vi "Update Dynamic Configurations.vi"(8 "error in":errorcluster, 10 "AsyncRequest":T2, 11 "Compiled.Settings in":T1) -> (0 "error out":errorcluster, 2 "Response Ref":refnum<queue>, 3 "Compiled.Settings out":T1)   [LabVIEW 2025, in "Runtime Configuration Support Inline Async Example Engine.lvlib"]
uses:
  Runtime Configuration Support Inline Async Example Engine.lvlib
  Shared/Compiled.Settings.ctl
  Shared/AsyncRequest.ctl
  Shared/Runtime Configuration Support Inline Async Example Shared.lvlib
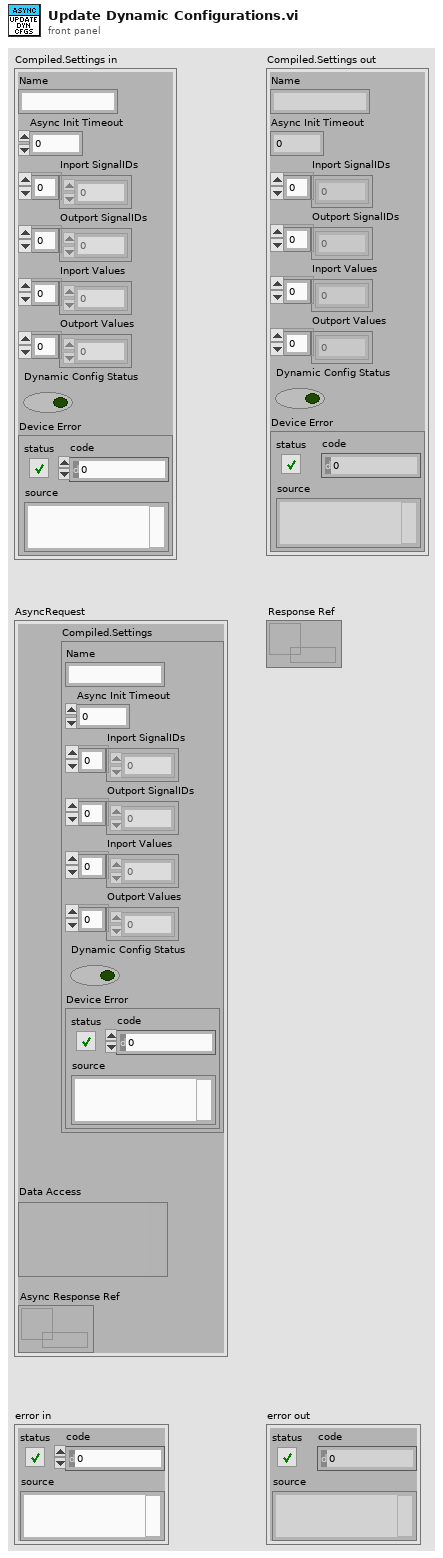
[diagram p1: front panel]
types:
  T1 = typedef "Runtime Configuration Support Inline Async Example Shared.lvlib/Compiled.Settings.ctl" = cluster{"Name":string, "Async Init Timeout":u16, "Inport SignalIDs":i32[], "Outport SignalIDs":i32[], "Inport Values":dbl[], "Outport Values":dbl[], "Dynamic Config Status":bool, "Device Error":errorcluster}
  T2 = typedef "Runtime Configuration Support Inline Async Example Engine.lvlib/AsyncRequest.ctl" = cluster{"Compiled.Settings":T1, "Data Access":variant, "Async Response Ref":refnum<queue>}
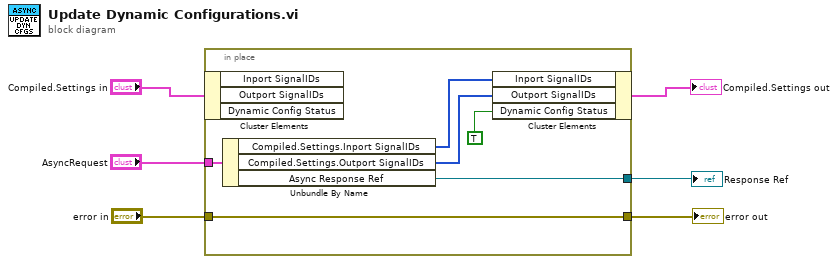
[diagram p0: block diagram]
diagram:
  n1 = in-place {
    in-place-border: "AsyncRequest" -> [w11]
    in-place-border: [w8] -> w2
    in-place-border: "error in" -> [w12]
    in-place-border: [w12] -> w5
    n2 = in-place-cluster #1("Compiled.Settings in") -> ()  [unwired: 3 out]
    n3 = Unbundle By Name(w11) -> ("Compiled.Settings.Inport SignalIDs"=w10:i32[], "Compiled.Settings.Outport SignalIDs"=w9:i32[], "Async Response Ref"=w8:refnum<queue>)
    n4 = in-place-cluster #1("Inport SignalIDs"=w10, "Outport SignalIDs"=w9, "Dynamic Config Status"=TRUE) -> (→"Compiled.Settings out":T1)
  }
  "Response Ref" <- w2
  "error out" <- w5
